vi "GA_WriteDataPathsToStr.vi"(8 "GA Metaparameters in":T1={"Training Data Path"=path "", "Test Data Path"=path "", "True Labels for Test Trials"=path "", "ClassifierType"=enum."Multilayer perceptron", "SVM Options"={"Kernel"=enum."Linear", "Degree"=0, "Gamma"=0.0, "Coefficient"=0.0, "Sigma"=0.0, "Cache(MB)"=0.0}, "GA Parameters"={"Population size"=0, "Generations no."=0, "Crossover probabality"=0.0, "Mutation mode"=enum."one-point, fixed rate", "Creep mutation"=FALSE, "Mutation rate"=0.0, "Min mutation rate"=0.0, "Max mutation rate"=0.0, "Relative fitness differential"=0.0, "Reproduction plan"=enum."Full generational replacement", "Elitism"=FALSE, "FeaturesPerChannel"=0}, "Use equal number of trials?"=FALSE, "Classifier Metaparameter"=5.0, "ClassifierQualityMeasure"=enum."Accuracy"} {"Classifier Metaparameter" min=0.0 max=100.0 step=0.1 format="%#_2g"; "GA Parameters"."Relative fitness differential" min=0.0 max=1.0; "GA Parameters"."Max mutation rate" min=0.0 max=1.0; "GA Parameters"."Min mutation rate" min=0.0 max=1.0; "GA Parameters"."Mutation rate" min=0.0 max=1.0; "GA Parameters"."Crossover probabality" min=0.0 max=1.0; "GA Parameters"."Generations no." min=1; "GA Parameters"."Population size" min=1}, 11 "String Ref in":refnum<vi>) -> (0 "error out":errorcluster, 2 "String out":string, 3 "String Ref out":refnum<vi>)   [LabVIEW 2016, in "GA.lvlib"]
uses:
  GA_metaParameters.ctl
  4. Accuracy Assessment for EEG Classification/_vlib/CU_ClassifierTypes.ctl
  <vilib>/vision/Classification.llb/IMAQ SVM Kernel Options.ctl
  GA_tParameters.ctl
  4. Accuracy Assessment for EEG Classification/_vlib/CU_ClassifierQualityMeasure.ctl
  GA.lvlib
  4. Accuracy Assessment for EEG Classification/Classifier.lvlib
panel:
  # "This VI is a part of BCI Design library, http://www.ru-bci.org \nCopyright © 2020, Sotnikov Peter, All rights reserved. License: CC BY-NC 4.0"
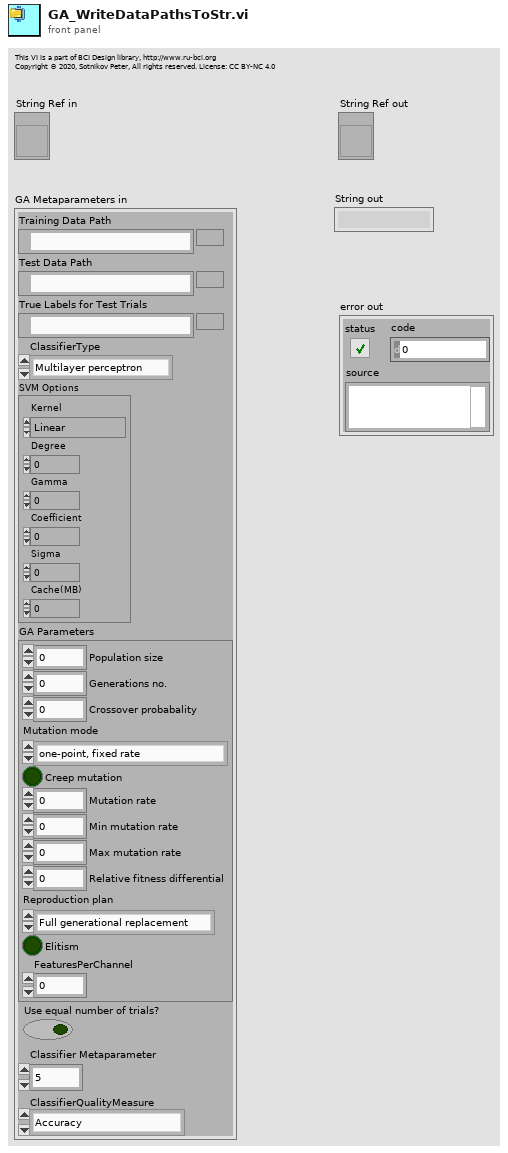
[diagram p1: front panel]
types:
  T1 = typedef "GA.lvlib/GA_metaParameters.ctl" = cluster{"Training Data Path":path, "Test Data Path":path, "True Labels for Test Trials":path, "ClassifierType":T2, "SVM Options":T3, "GA Parameters":T4, "Use equal number of trials?":bool, "Classifier Metaparameter":dbl, "ClassifierQualityMeasure":T5}
  T2 = typedef "Classifier.lvlib/CU_ClassifierTypes.ctl" = enum16{"Multilayer perceptron", "k NN Classifier", "SVM Committee", "Mahalanobis distance", "SVM Classifier"}
  T3 = typedef "IMAQ SVM Kernel Options.ctl" = cluster{"Kernel":enum32{"Linear", "Polynomial", "Gaussian", "RBF"}, "Degree":i32, "Gamma":dbl, "Coefficient":dbl, "Sigma":dbl, "Cache(MB)":dbl}
  T4 = typedef "GA.lvlib/GA_tParameters.ctl" = cluster{"Population size":i32, "Generations no.":i32, "Crossover probabality":dbl, "Mutation mode":enum16{"one-point, fixed rate", "one-point, fitness-adjustable rate", "one-point, distance-adjustable rate"}, "Creep mutation":bool, "Mutation rate":dbl, "Min mutation rate":dbl, "Max mutation rate":dbl, "Relative fitness differential":dbl, "Reproduction plan":enum16{"Full generational replacement", "Steady-state-replace-random", "Steady-state-replace-worst"}, "Elitism":bool, "FeaturesPerChannel":i32}
  T5 = typedef "Classifier.lvlib/CU_ClassifierQualityMeasure.ctl" = enum16{"Accuracy", "Cohen's kappa"}
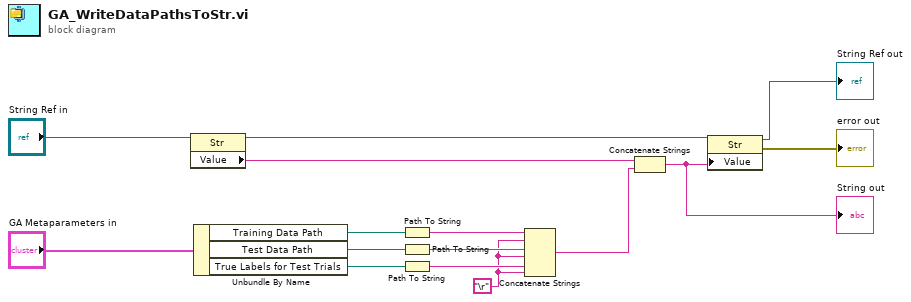
[diagram p0: block diagram]
diagram:
  w8 = "\r"
  n1 = property class="Str"(reference="String Ref in") -> (reference out=w6:refnum<vi>, "Value"=w5:string)  [unwired: 1 in, 1 out]
  n2 = Unbundle By Name("GA Metaparameters in") -> ("Training Data Path"=w14:path, "Test Data Path"=w13:path, "True Labels for Test Trials"=w12:path)
  n3 = Path To String(path=w14) -> (string=w11:string)
  n4 = Path To String(path=w13) -> (string=w10:string)
  n5 = Path To String(path=w12) -> (string=w9:string)
  n6 = Concatenate Strings(w11, w8, w10, w8, w9, w8) -> (w4:string)
  n7 = Concatenate Strings(w5, w4) -> (w3:string)
  "String out" <- w3
  n8 = property class="Str"(reference=w6, "Value"=w3) -> (reference out=→"String Ref out":refnum<vi>, error out=→"error out":errorcluster)  [unwired: 1 in]
